vi "ellipse graph.vi"(0 "# of points":i32, 2 "Avg Variation":cluster{"Avg X Var":dbl, "Avg Y Var":dbl}, 4 "Center":cluster{"Avg X Var":dbl, "Avg Y Var":dbl}) -> (7 "ellipse graph":cluster{dbl[], dbl[]})   [LabVIEW 2013]
uses:
  <vilib>/Analysis/1siggen.llb/Ramp Pattern by Samples.vi
  <vilib>/Analysis/NI_AALBase.lvlib
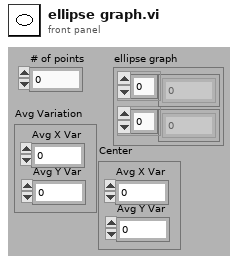
[diagram p1: front panel]
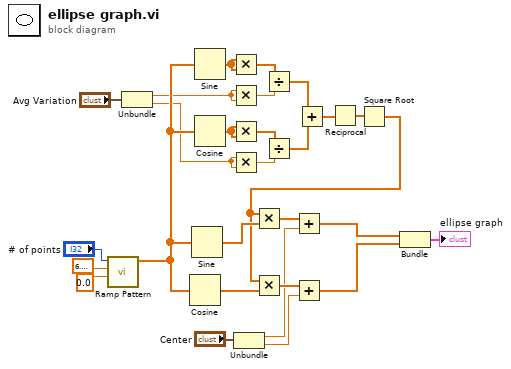
[diagram p0: block diagram]
diagram:
  n1 = call-poly <vilib>:"Ramp Pattern.vi"("start"=0.0, "end"=6.283185307179586, "samples"="# of points") -> ("Ramp Pattern"=w14:dbl[])  [unwired: 7 in, 1 out]
  n2 = Unbundle("Avg Variation") -> ("Avg X Var"=w10:dbl, "Avg Y Var"=w9:dbl)
  n3 = Cosine(x=w14) -> (cos(x)=w24:dbl[])
  n4 = Sine(x=w14) -> (sin(x)=w25:dbl[])
  n5 = Sine(x=w14) -> (sin(x)=w22:dbl[])
  n6 = Cosine(x=w14) -> (cos(x)=w18:dbl[])
  n7 = Multiply(x=w22, y=w22) -> (x*y=w21:dbl[])
  n8 = Multiply(x=w10, y=w10) -> (x*y=w20:dbl)
  n9 = Multiply(x=w18, y=w18) -> (x*y=w17:dbl[])
  n10 = Multiply(x=w9, y=w9) -> (x*y=w19:dbl)
  n11 = Unbundle("Center") -> ("Avg X Var"=w2:dbl, "Avg Y Var"=w1:dbl)
  n12 = Divide(x=w21, y=w20) -> (x/y=w15:dbl[])
  n13 = Divide(x=w17, y=w19) -> (x/y=w16:dbl[])
  n14 = Add(x=w16, y=w15) -> (x+y=w13:dbl[])
  n15 = Reciprocal(x=w13) -> (1/x=w12:dbl[])
  n16 = Square Root(x=w12) -> (sqrt(x)=w11:dbl[])
  n17 = Multiply(x=w11, y=w25) -> (x*y=w6:dbl[])
  n18 = Multiply(x=w11, y=w24) -> (x*y=w4:dbl[])
  n19 = Add(x=w6, y=w2) -> (x+y=w5:dbl[])
  n20 = Add(x=w4, y=w1) -> (x+y=w3:dbl[])
  n21 = Bundle(w5, w3) -> (→"ellipse graph":cluster{dbl[], dbl[]})  [unwired: 1 out]
